vi "solar_write QTimerStart.vi"(8 "error in (no error)":errorcluster, 10 "QTimer":string, 11 "solar in":refnum<class "solar.lvclass">) -> (0 "error out":errorcluster, 3 "solar out":refnum<class "solar.lvclass">)   [LabVIEW 2018, in "solar.lvclass"]
doc: "This starts the specified QTimer."
uses:
  solar.lvclass
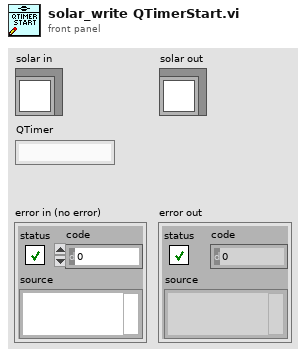
[diagram p1: front panel]
types:
  T1 = typedef "solar_ctl SOLAR Refnum.ctl" = refnum<k1>
  T2 = typedef "solar_ctl SOLAR Global.ctl" = cluster{"Targets":T3[], "AppDir":path, "solar.ini":path, "ConfigsDir":path, "CosmosDir":path, "LogsDir":path, "ExePath":path, "ExeVersion":string, "PartNum":string, "AppSetup":string, "Title":string, "Main.ini":path, "Temp.ini":path, "vSOLAR":string, "Splash.png":string, "SplashWait":i32, "SOLARUE":refnum<user-event>, "VoyagerRefnum":T4, "QTimerRefnum":T5}
  T3 = typedef "solar_ctl Target Global.ctl" = cluster{"Target":string, "Q":refnum<queue>, "UE":refnum<user-event>, "VI":refnum<vi>, "Menu":refnum<k9>, "Data":refnum<data-value>, "Attributes":variant}
  T4 = typedef "solar_voy_ctl Voyager Refnum.ctl" = refnum<k1>
  T5 = typedef "solar_qtimer_ctl Refnum.ctl" = refnum<k1>
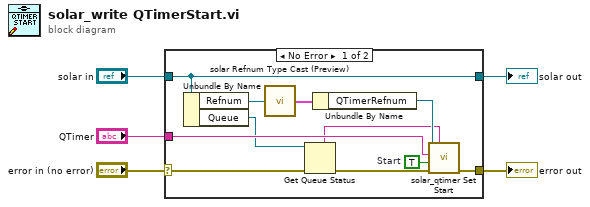
[diagram p0: block diagram]
diagram:
  n1 = case shown="No Error" "error in (no error)" {
    selector: "error in (no error)" -> [w9 w18]
    tunnel: "solar in" -> [w14 w17]
    tunnel: [w13 w18] -> w4
    tunnel: [w14 w17] -> w2
    tunnel: "QTimer" -> [w11 _]
    frame No Error {
      w10 = TRUE  # Start
      n2 = Unbundle By Name(w14) -> ("Refnum"=w16:T1, "Queue"=w7:refnum<queue>)
      n3 = call "solar Refnum Type Cast (Preview).vi"("Refnum"=w16) -> ("SOLAR"=w15:T2)  [unwired: 8 in]
      n4 = Get Queue Status(queue=w7, error in (no error)=w9) -> (queue name=w6:string, error out=w8:errorcluster)  [unwired: 1 in, 6 out]
      n5 = Unbundle By Name(w15) -> ("QTimerRefnum"=w12:T5)
      n6 = call "solar_qtimer Set Start.vi"("Target Name"=w6, "error in (no error)"=w8, "Start (F = Stop)"=w10, "QTimer Name"=w11, "QTimer Refnum in"=w12) -> ("error out"=w13:errorcluster)  [unwired: 5 in, 1 out]
    }
    frame Error {
    }
  }
  "error out" <- w4
  "solar out" <- w2
